vi "DetectPCIDGs and Initialize System.vi"(8 "error in (no error)":errorcluster, 10 "Calibrate?":bool, 11 "BME_DG_System in":refnum<class "BME_DG_System.lvclass">) -> (0 "error out":errorcluster, 2 "NumberOfCards":i32, 3 "BME_DG_System out":refnum<class "BME_DG_System.lvclass">)   [LabVIEW 2009, in "POLARIS BME DG.lvlib" / "BME_DG_System.lvclass"]
uses:
  BME_DG_System.lvclass
  BME_DG_System.lvclass/BME_DG_System.ctl
  POLARIS BME DG.lvlib
panel:
  in  "p_Error in":i32
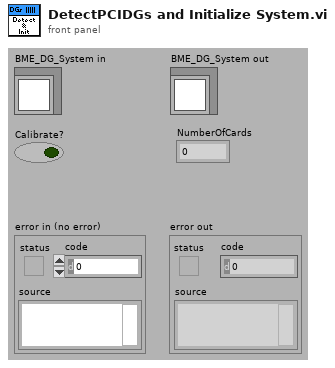
[diagram p1: front panel]
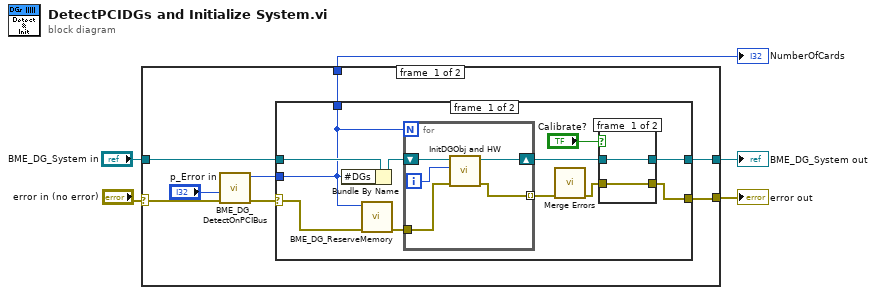
[diagram p0: block diagram]
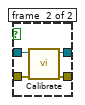
[diagram p2: hidden frame]
diagram:
  n1 = case shown="No Error" "error in (no error)" {
    selector: "error in (no error)" -> [w12 w39]
    tunnel: [w7 w39] -> w4
    tunnel: [w10 w38] -> w2
    tunnel: "BME_DG_System in" -> [w13 w38]
    tunnel: [w6 _] -> w1
    frame #0 {
      n2 = call "BME_DG_DetectOnPCIBus.vi"("error in (no error)"=w12, "p_Error in"="p_Error in") -> ("error out"=w8:errorcluster, "NumberOfCards"=w9:i32)  [unwired: 7 in, 1 out]
      n3 = case shown="No Error" w8 {
        selector: w8 -> [w22 w36]
        tunnel: w13 -> [w24 w37]
        tunnel: [w19 w37] -> w10
        tunnel: w9 -> [w14 _]
        tunnel: [w15 w36] -> w7
        tunnel: [w14 _] -> w6
        frame #0 {
          n4 = Bundle By Name(cluster=w24, "#DGs"=w14) -> (w23:refnum<class "BME_DG_System.lvclass">)
          n5 = call "BME_DG_ReserveMemory.vi"("error in (no error)"=w22, "Number of Cards"=w14) -> ("error out"=w21:errorcluster)  [unwired: 8 in, 1 out]
          n6 = for {
            N: w14 -> [_]
            shift-right: [w34] -> w20
            shift-left: w23 -> [w33]
            tunnel: w21 -> [w32]
            tunnel: [w31] -> w17 mode=indexing
            i -> [w35]
            n7 = call "InitDGObj and HW.vi"("error out"=w32, "DGNr"=w35, "BME_DG_System in"=w33) -> ("error IO"=w31:errorcluster, "BME_DG_System Out"=w34:refnum<class "BME_DG_System.lvclass">)  [unwired: 3 in]
          }
          n8 = call <vilib>:"Merge Errors.vi"("error array in"=w17) -> ("error out"=w18:errorcluster)  [unwired: 6 in]
          n9 = case shown="True" "Calibrate?" {
            tunnel: w20 -> [w26 w30]
            tunnel: [w26 w29] -> w19
            tunnel: w18 -> [w25 w28]
            tunnel: [w25 w27] -> w15
            frame #0 {
            }
            frame #1 {
              n10 = call "Calibrate.vi"("error in (no error)"=w28, "BME_DG_System in"=w30) -> ("error out"=w27:errorcluster, "BME_DG_System out"=w29:refnum<class "BME_DG_System.lvclass">)  [unwired: 8 in]
            }
          }
        }
        frame #1 {
        }
      }
    }
    frame #1 {
    }
  }
  "error out" <- w4
  "BME_DG_System out" <- w2
  "NumberOfCards" <- w1
